vi "solar_addon EnQ.vi"(11 "Variant":variant) -> (0 "error out":errorcluster)   [LabVIEW 2018]
doc: "This enqueues a message to a target specified by the <b>Command String</b> formatted as:\n\n<b>TARGET:CMD{\nTYPE:VALUE,\nTYPE:\"VALUE\"}</b>\n\n<b>TYPE</b>= I8, I16, I32, I64, U8, U16, U32, U64, U8_ENUM, U16_ENUM, U32_ENUM, SGL, DBL, BOOL, STR, PATH, TIME\n<type>_1D:\"<comma delimited>\"\n<type>_2D:\"<comma & line feed delimited>\"\nDefine enum items after the TYPE. Ex: '<b>U8_ENUM[i0,i1,i2]:VALUE</b>' where VALUE is <numeric> or <string>\n\nMyTarget:MyCMD{\nI32:-1234,\nSTR:\"Hello World\",\nU16_ENUM[Item1,Item2,Item3]:\"Item2\",\nBOOL:true,\nTIME:\"yyyy-mm-dd_hh:mm:ss.uuuuuu\",\nPATH:\"C:\\Data\\test.txt\",\nU8_2D:\"1,2,3\n4,5,6\"}"
uses:
  <vilib>/Utility/miscctls.llb/LVSelectionTypeDef.ctl
  solar/solar_ctl SOLAR Refnum.ctl
panel:
  in  "#":i32
  in  "Command List":u16(ring) items=["Select Command...", "TARGET:INITIALIZE{}", "TARGET:REGISTER{}", "TARGET:EXIT{}", "TARGET:CONNECT{}", "TARGET:DISCONNECT{}", "TARGET:READ{}", "TARGET:EXAMPLE{I32:123,STR:'Hello World',U16_ENUM|item1|item2:'item2'}", "TARGET:EXAMPLE2{U16_2D:'1,2,3;4,5,6'}"]
  out "Received Time":string
  out "Command":string
  out "Target":string
  out "CMD_DATA":variant caption="Command Variant"
  out "Status":string
  in  "Command String":string caption="Command String (Ctrl-H)"
  in  "Clear":bool
  in  "Send":bool
  in  "Handshake?":bool
  in  "Handshake Timeout":u32=60000 format="%d ms"
  in  "Priority":enum8{"Normal", "Priority", "IgnoreIfExists"}(ring)
  out "TLM_DATA":variant caption="Telemetry Data"
  out "Error":errorcluster
  out "TLM":string caption="Telemetry"
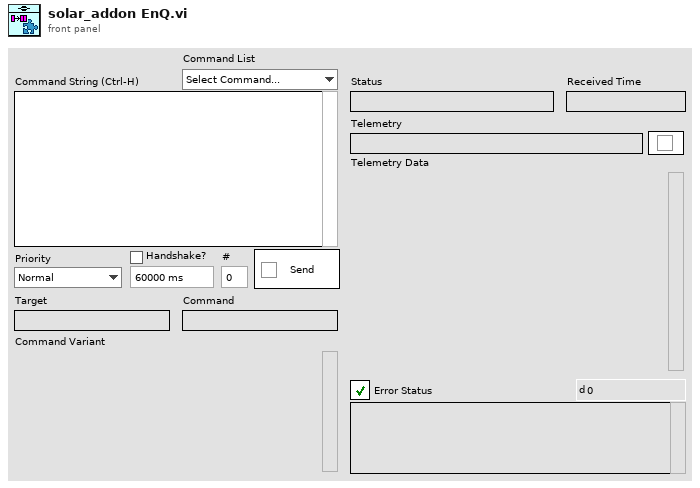
[diagram p1: front panel]
types:
  T1 = typedef "solar_ctl SOLAR Refnum.ctl" = refnum<k1>
  T2 = typedef "LVSelectionTypeDef.ctl" = cluster{"Selection Start":u32, "Selection End":u32}
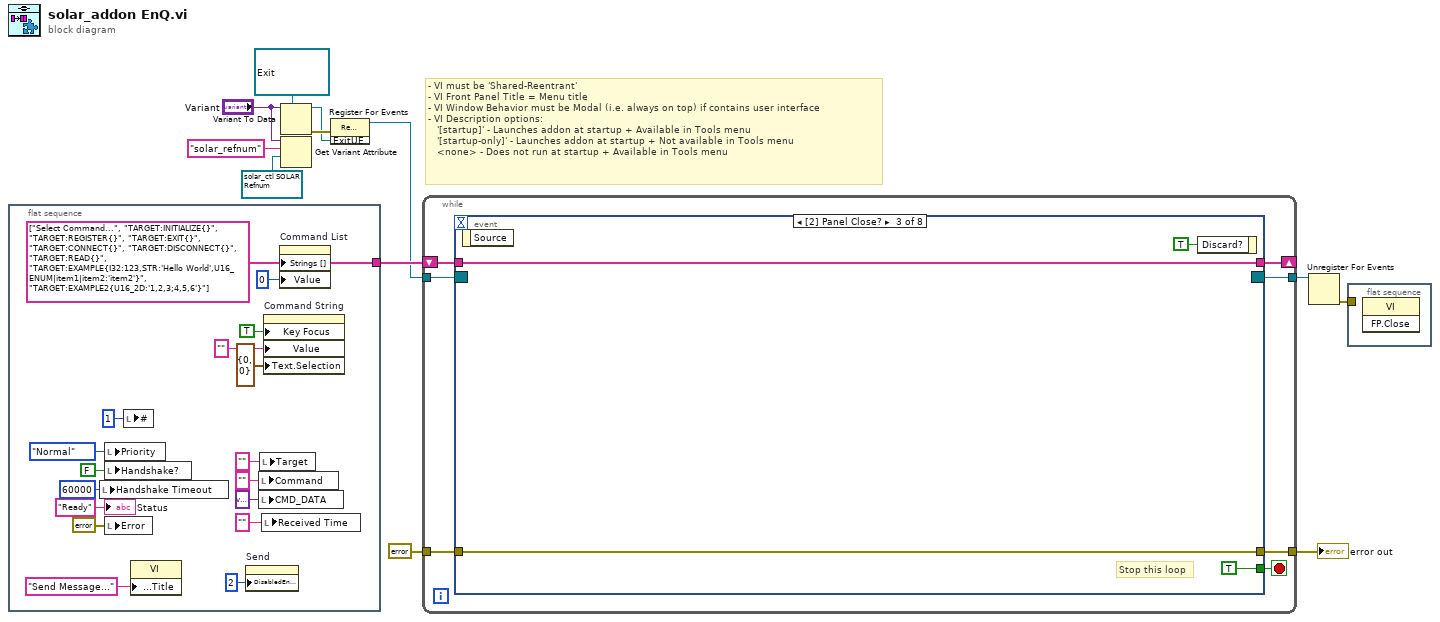
[diagram p0: block diagram]
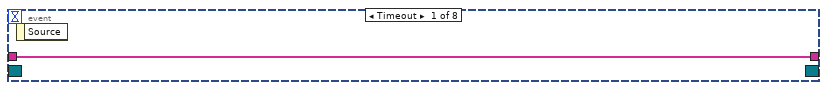
[diagram p2: hidden frame]
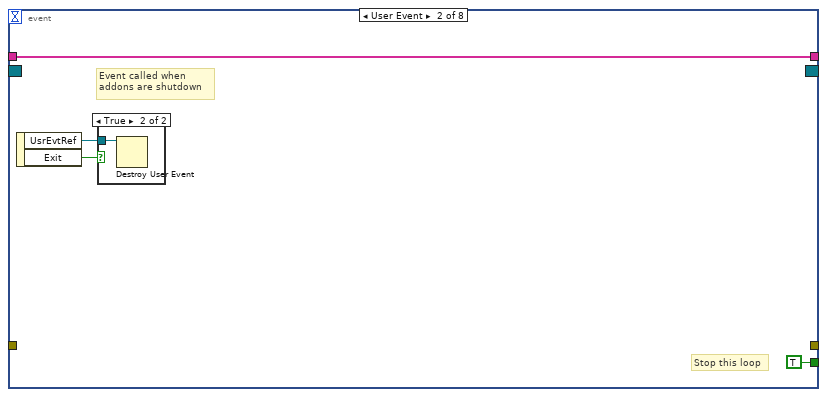
[diagram p3: hidden frame]
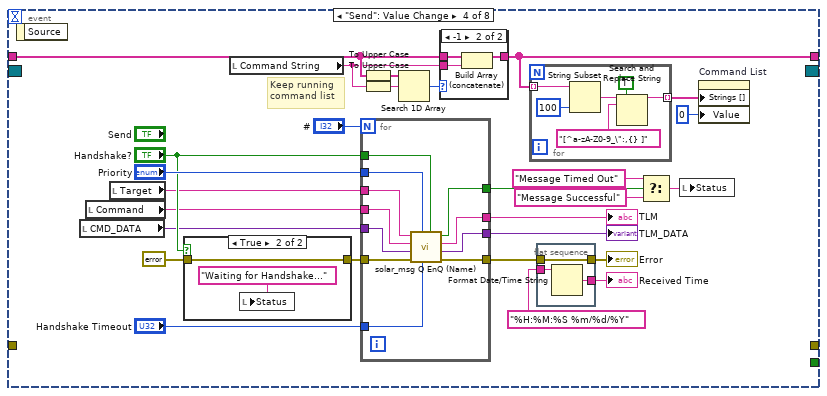
[diagram p5: hidden frame]
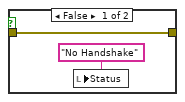
[diagram p7: hidden frame]
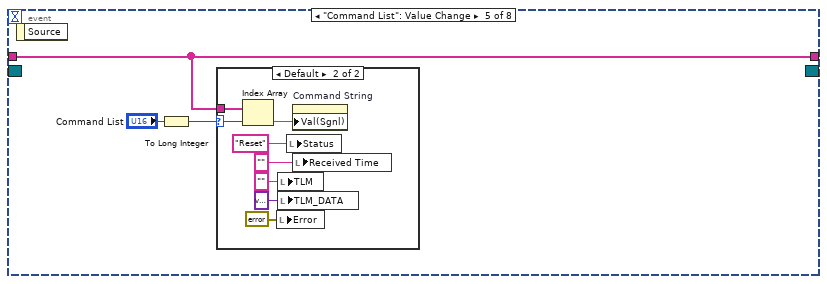
[diagram p8: hidden frame]
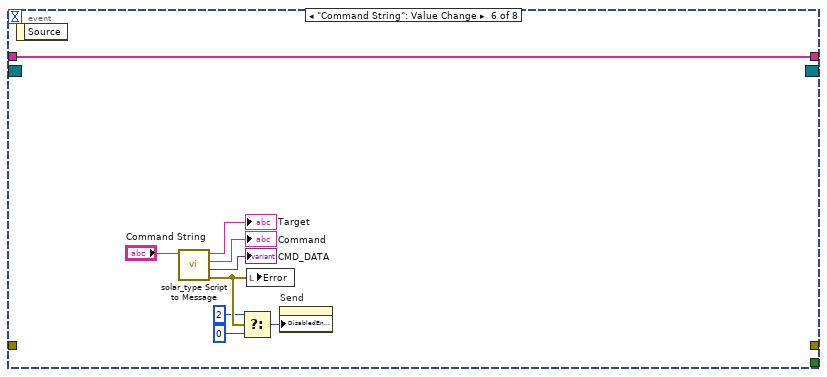
[diagram p10: hidden frame]
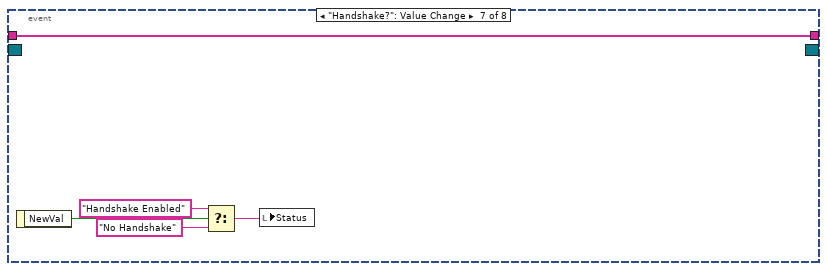
[diagram p11: hidden frame]
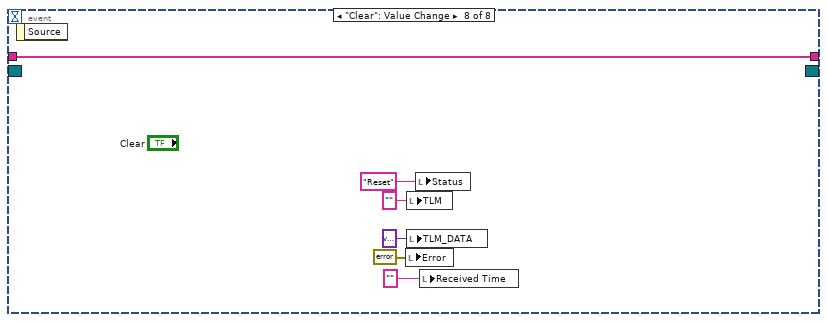
[diagram p12: hidden frame]
diagram:
  w7 = T1 refnum items=["solar"] ("SOLAR Refnum")
  # "- VI must be 'Shared-Reentrant'\n- VI Front Panel Title = Menu title\n- VI Window Behavior must be Modal (i.e. always on top) if contains user interface\n- VI Description options:\n   '[startup]' - Launches addon at startup + Available in Tools menu\n   '[startup-only]' - Launches addon at startup + Not available in Tools menu\n   <none> - Does not run at startup + Available in Tools menu"
  n1 = flat-sequence {
    tunnel: [w14] -> w12
    frame #0 {
      w14 = string[] ["Select Command...", "TARGET:INITIALIZE{}", "TARGET:REGISTER{}", "TARGET:EXIT{}", "TARGET:CONNECT{}", "TARGET:DISCONNECT{}", "TARGET:READ{}", "TARGET:EXAMPLE{I32:123,STR:'Hello World',U16_ENUM|item1|item2:'item2'}", "TARGET:EXAMPLE2{U16_2D:'1,2,3;4,5,6'}"] ("Strings []")
      n2 = local write "Handshake Timeout"(u32 60000 ("HS_Timeout")) -> ()
      n3 = local write "Priority"(enum8{"Normal", "Priority", "IgnoreIfExists"}."Normal" ("Priority")) -> ()
      n4 = local write "Handshake?"(FALSE ("Handshake?")) -> ()
      n5 = local write "Error"(errorcluster {"status"=FALSE, "code"=0, "source"=""} ("Error")) -> ()
      n6 = local write "#"(1 ("#")) -> ()
      n7 = property class="VI"("Front Panel.Title"="Send Message..." ("Front Panel Window:Title")) -> ()  [unwired: 2 in, 2 out]
      n8 = property on="Send" class="Bool"("DisabledEnum"=u8 2) -> ()  [unwired: 2 in, 2 out]
      n9 = local write "Command"("" ("Command")) -> ()
      n10 = local write "CMD_DATA"(variant ("CMD_DATA")) -> ()
      n11 = local write "Target"("" ("Target")) -> ()
      n12 = local write "Received Time"("" ("Telemetry Received")) -> ()
      n13 = property on="Command String" class="Str"("Key Focus"=TRUE, "Value"="" ("CMD_DATA_Packet"), "Text.Selection"=T2 {"Selection Start"=0, "Selection End"=0}) -> ()  [unwired: 2 in, 2 out]
      n14 = property on="Command List" class="Ring (strict)"("Strings []"=w14, "Value"=u16 0) -> ()  [unwired: 2 in, 2 out]
      "Status" <- "Ready" ("HS_Status")
    }
  }
  n15 = Variant To Data(type=refnum<user-event> refnum ("ExitUE"), Variant="Variant") -> (data=w10:refnum<user-event>, error out=w11:errorcluster)  [unwired: 1 in]
  n16 = Get Variant Attribute(Variant="Variant", name="solar_refnum", default value (empty Variant)=w7) -> ()  [unwired: 1 in, 4 out]
  n17 = register-events(error in=w11, w10) -> (reference out=w8:refnum<event-registration>)  [unwired: 1 in, 1 out]
  n18 = while {
    shift-right: [w35] -> _
    shift-left: w12 -> [w36]
    tunnel: w8 -> [w34]
    tunnel: [w32] -> w4
    tunnel: [w31] -> w2
    tunnel: errorcluster {"status"=FALSE, "code"=0, "source"=""} ("error in (no error)") -> [w30]
    stop <- w33 stop-if-true
    n19 = event shown="[2] Panel Close?" {
      selector: w34 -> [_ _ _ _ _ _ _ _]
      dyn-events: [_ _ _ _ _ _ _ _] -> w32
      timeout: _ -> [_ _ _ _ _ _ _ _]
      tunnel: [_ TRUE TRUE _ _ _ _ _] -> w33
      tunnel: w36 -> [w37 w41 w45 w58 w103 w113 w122 w127]
      tunnel: [w37 w41 w45 w54 w103 w113 w122 w127] -> w35
      tunnel: [_ _ w43 _ _ _ _ _] -> w31
      tunnel: w30 -> [_ _ w43 _ _ _ _ _]
      event Timeout {
        n20 = event-data() -> ()  [unwired: 1 in, 1 out]
      }
      event User Event {
        # "Stop this loop"
        # "Event called when\naddons are shutdown"
        n21 = event-data() -> ("UsrEvtRef"=w39:refnum<user-event>, "Exit"=w38:bool)  [unwired: 1 in]
        n22 = case shown="True" w38 {
          tunnel: w39 -> [_ w42]
          frame False {
          }
          frame True {
            n23 = Destroy User Event(user event=w42) -> ()  [unwired: 1 in, 1 out]
          }
        }
      }
      event Panel Close? {
        # "Stop this loop"
        n24 = event-data() -> ()  [unwired: 1 in, 1 out]
        n25 = event-data("Discard?"=TRUE) -> ()  [unwired: 1 in, 1 out]
      }
      event "Send": Value Change {
        # "Keep running\ncommand list"
        n26 = event-data() -> ()  [unwired: 1 in, 1 out]
        n27 = local read "CMD_DATA"() -> (w62:variant)
        n28 = local read "Command"() -> (w66:string)
        n29 = local read "Target"() -> (w67:string)
        n30 = case shown="True" "Handshake?" {
          tunnel: [w95 w97] -> w64
          tunnel: errorcluster {"status"=FALSE, "code"=0, "source"=""} ("error out") -> [w95 w97]
          frame False {
            n31 = local write "Status"("No Handshake" ("HS_Status")) -> ()
          }
          frame True {
            n32 = local write "Status"("Waiting for Handshake..." ("HS_Status")) -> ()
          }
        }
        n33 = local read "Command String"() -> (w55:string)
        n34 = for {
          N: "#" -> [_]
          tunnel: "Handshake Timeout" -> [w84]
          tunnel: "Priority" -> [w83]
          tunnel: w67 -> [w79]
          tunnel: w64 -> [w76]
          tunnel: [w77] -> w65
          tunnel: w62 -> [w75]
          tunnel: [w82] -> w71
          tunnel: w66 -> [w78]
          tunnel: [w81] -> w70
          tunnel: "Handshake?" -> [w80]
          tunnel: [w74] -> w51
          n35 = call "solar_msg Q EnQ (Name).vi"("Handshake? (F)"=w80, "HS Timeout ms (60000)"=w84, "Priority (Normal)"=w83, "error in (no error)"=w76, "CMD_DATA"=w75, "CMD"=w78, "Target"=w79) -> ("error out"=w77:errorcluster, "TLM_DATA"=w82:variant, "TLM"=w81:string, "TLM Timed Out?"=w74:bool)  [unwired: 1 in]
        }
        "TLM_DATA" <- w71
        "TLM" <- w70
        n36 = To Upper Case(1:w58) -> (0:w57:string[])
        n37 = To Upper Case(1:w55) -> (0:w56:string)
        n38 = Search 1D Array(1D array=w57, element=w56) -> (index of element=w59:i32)  [unwired: 1 in]
        n39 = case shown="-1" w59 {
          tunnel: [w91 w93] -> w54
          tunnel: w58 -> [w91 w94]
          tunnel: w55 -> [_ w92]
          frame Default {
          }
          frame -1 {
            n40 = Build Array (concatenate)(w94, w92) -> (w93:string[])
          }
        }
        n41 = for {
          tunnel: w54 -> [w90] mode=indexing
          tunnel: [w85] -> w48 mode=indexing
          n42 = String Subset(string=w90, length (rest)=100 ("length (rest)")) -> (substring=w86:string)  [unwired: 1 in]
          n43 = Search and Replace String(replace all?=TRUE, input string=w86, search string="[^a-zA-Z0-9_\":,{} ]") -> (result string=w85:string)  [unwired: 5 in, 3 out]
        }
        n44 = flat-sequence {
          tunnel: [w101] -> w69
          tunnel: w65 -> [w101]
          tunnel: [w100] -> w61
          tunnel: "%H:%M:%S %m/%d/%Y" ("time format string (%c)") -> [w99]
          frame #0 {
            n45 = Format Date/Time String(time format string (%c)=w99) -> (date/time string=w100:string)  [unwired: 2 in]
          }
        }
        n46 = Select(t="Message Timed Out" ("HS_Status"), s=w51, f="Message Successful" ("HS_Status")) -> (s? t:f=w49:string)
        n47 = local write "Status"(w49) -> ()
        n48 = property on="Command List" class="Ring (strict)"("Strings []"=w48, "Value"=u16 0) -> ()  [unwired: 2 in, 2 out]
        "Error" <- w69
        "Received Time" <- w61
      }
      event "Command List": Value Change {
        n49 = event-data() -> ()  [unwired: 1 in, 1 out]
        n50 = To Long Integer(number="Command List") -> (32bit integer=w102:i32)
        n51 = case shown="Default" w102 {
          selector: w102 -> [_ w105]
          tunnel: w103 -> [_ w112]
          frame 0 {
          }
          frame Default {
            n52 = Index Array(array=w112, index=w105) -> (element=w111:string)
            n53 = local write "Error"(errorcluster {"status"=FALSE, "code"=0, "source"=""} ("Error")) -> ()
            n54 = local write "TLM"("" ("TLM")) -> ()
            n55 = local write "TLM_DATA"(variant ("TLM_DATA")) -> ()
            n56 = local write "Status"("Reset" ("HS_Status")) -> ()
            n57 = property on="Command String" class="Str"("Val(Sgnl)"=w111) -> ()  [unwired: 2 in, 2 out]
            n58 = local write "Received Time"("" ("Message Completed")) -> ()
          }
        }
      }
      event "Command String": Value Change {
        n59 = event-data() -> ()  [unwired: 1 in, 1 out]
        n60 = call "solar_type Script to Message.vi"("Script String"="Command String") -> ("error out"=w117:errorcluster, "Data"=→"CMD_DATA":variant, "Packet"=→"Command":string, "Target"=→"Target":string)  [unwired: 5 in, 2 out]
        n61 = Select(t=u8 2, s=w117, f=u8 0) -> (s? t:f=w114:u8)
        n62 = local write "Error"(w117) -> ()
        n63 = property on="Send" class="Bool"("DisabledEnum"=w114) -> ()  [unwired: 2 in, 2 out]
      }
      event "Handshake?": Value Change {
        n64 = event-data() -> ("NewVal"=w126:bool)  [unwired: 1 in]
        n65 = Select(t="Handshake Enabled" ("HS_Status"), s=w126, f="No Handshake" ("HS_Status")) -> (s? t:f=w123:string)
        n66 = local write "Status"(w123) -> ()
      }
      event "Clear": Value Change {
        n67 = event-data() -> ()  [unwired: 1 in, 1 out]
        n68 = local write "Error"(errorcluster {"status"=FALSE, "code"=0, "source"=""} ("Error")) -> ()
        n69 = local write "TLM"("" ("TLM")) -> ()
        n70 = local write "TLM_DATA"(variant ("TLM_DATA")) -> ()
        n71 = local write "Status"("Reset" ("HS_Status")) -> ()
        n72 = local write "Received Time"("" ("Telemetry Received")) -> ()
      }
    }
  }
  "error out" <- w2
  n73 = Unregister For Events(event registration refnum=w4) -> (error out=w3:errorcluster)  [unwired: 1 in]
  n74 = flat-sequence {
    tunnel: w3 -> [_]
    frame #0 {
      n75 = invoke class="VI" method="FP.Close"() -> ()  [unwired: 3 in, 3 out]
    }
  }
